vi "pume_read.vi"() -> ()   [LabVIEW 2013]
panel:
  out "Registers":u16[](array[numeric]) caption="Registers to Write" format="%x"
  in  "Q":u8=128
  in  "Address":u16=9600
  in  "Serial Parameters":T1={"Mode"=enum."RTU", "Slave Address"=1} {"Slave Address" format="%x"}
  in  "Timeout":u32=10000
  in  "Flow Control":u16(ring) items=["None", "XON/XOFF", "RTS/CTS", "XON/XOFF & RTS/CTS", "DTR/DSR", "XON/XOFF & DTR/DSR"]
  in  "Parity":u16(ring) items=["None", "Odd", "Even", "Mark", "Space"]
  in  "Baud Rate":u32=9600
  in  "Port":refnum<visa-resource-name>
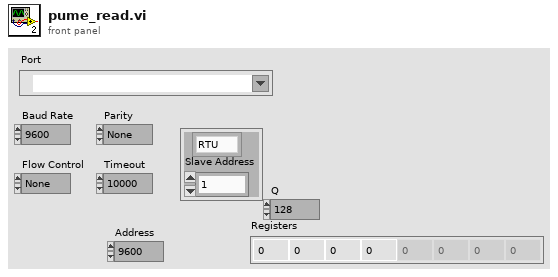
[diagram p1: front panel]
types:
  T1 = cluster{"Mode":enum16{"RTU", "ASCII"}, "Slave Address":u8}
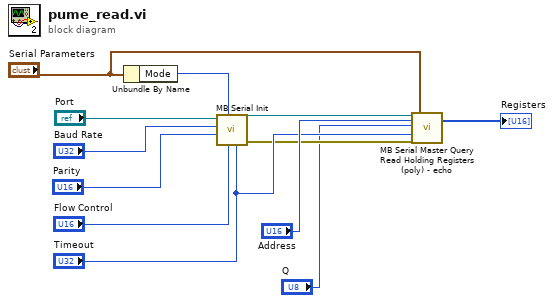
[diagram p0: block diagram]
diagram:
  n1 = Unbundle By Name("Serial Parameters") -> ("Mode"=w8:enum16{"RTU", "ASCII"})
  n2 = call "MB Serial Init.vi"("Timeout"="Timeout", "Flow Control"="Flow Control", "Mode"=w8, "Parity"="Parity", "Baud Rate"="Baud Rate", "VISA resource name"="Port") -> ("error out"=w3:errorcluster, "VISA resource name out"=w6:refnum<visa-resource-name>)  [unwired: 1 in, 3 out]
  n3 = call "MB Serial Master Query Read Holding Registers (poly) - echo.vi"("VISA resource name"=w6, "Starting Address"="Address", "Quantity"="Q", "Timeout"="Timeout", "error in"=w3, "Serial Parameters"="Serial Parameters") -> ("Holding Registers"=→"Registers":u16[])  [unwired: 10 in, 3 out]
